vi "Last_Window.vi"(0 "Produced_Time":timestamp[](array[timestamp]), 4 "Windows_Last_Index":i32, 5 "Window_Spark_Rate_IN":dbl[](array[numeric]), 6 "Threshold [uA]":dbl=0.05 min=0.0001 max=50.0 format="%#_13g", 7 "Window_Median_IN":dbl[](array[numeric]), 9 "Window_Avg_IN":dbl[](array[numeric]), 10 "Window size [min]":i64=5 min=1 max=180, 11 "Origin_Time":timestamp[](array[timestamp]), 15 "Origin_Current_IN":dbl[](array[numeric])) -> (1 "Time_Out":timestamp[](array[timestamp]), 3 "Window_Avg_OUT":dbl[](array[numeric]), 8 "Window_Median_OUT":dbl[](array[numeric]), 12 "Last_Window":cluster{timestamp[], dbl[]}(graph), 14 "Window_Spark_Rate_OUT":dbl[](array[numeric]))   [LabVIEW 2018]
uses:
  <vilib>/Analysis/NI_AALBase.lvlib
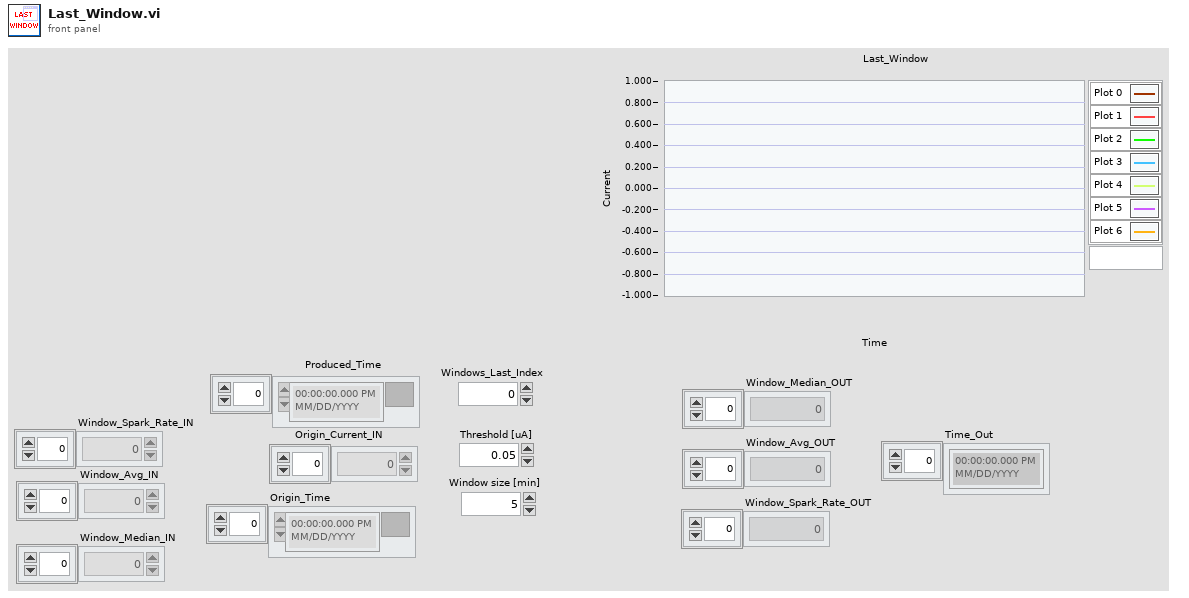
[diagram p1: front panel]
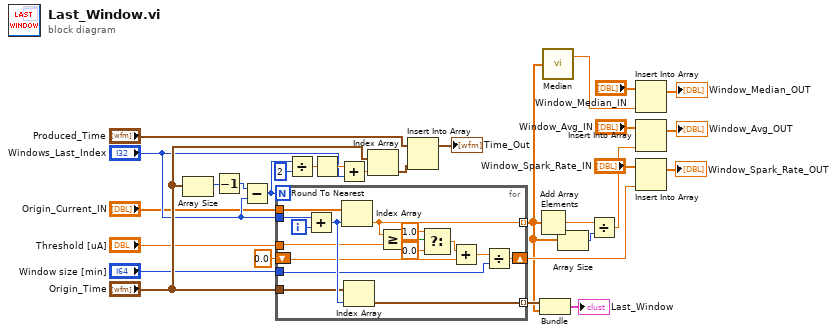
[diagram p0: block diagram]
diagram:
  n1 = Array Size(array="Origin_Time") -> (size(s)=w29:i32)
  n2 = Decrement(x=w29) -> (x-1=w18:i32)
  n3 = Subtract(x=w18, y="Windows_Last_Index") -> (x-y=w25:i32)
  n4 = for {
    N: w25 -> [_]
    tunnel: "Origin_Current_IN" -> [w35]
    tunnel: "Windows_Last_Index" -> [w46]
    tunnel: [w36] -> w2 mode=indexing
    tunnel: "Origin_Time" -> [w43]
    tunnel: [w42] -> w28 mode=indexing
    shift-right: [w34] -> w21
    shift-left: 0.0 -> [w33]
    tunnel: "Threshold [uA]" -> [w32]
    tunnel: "Window size [min]" -> [w31]
    i -> [w45]
    n5 = Add(x=w46, y=w45) -> (x+y=w44:i32)
    n6 = Index Array(array=w35, index=w44) -> (element=w36:dbl)
    n7 = Index Array(array=w43, index=w44) -> (element=w42:timestamp)
    n8 = Greater Or Equal?(x=w36, y=w32) -> (x >= y?=w40:bool)
    n9 = Select(t=1.0, s=w40, f=0.0) -> (s? t:f=w41:dbl)
    n10 = Add(x=w41, y=w33) -> (x+y=w39:dbl)
    n11 = Divide(x=w39, y=w31) -> (x/y=w34:dbl)
  }
  n12 = Divide(x=w25, y=2) -> (x/y=w24:dbl)
  n13 = Round To Nearest(number=w24) -> (nearest integer value=w23:dbl)
  n14 = Add(x=w23, y="Windows_Last_Index") -> (x+y=w22:dbl)
  n15 = Index Array(array="Origin_Time", index=w22) -> (element=w19:timestamp)
  n16 = Insert Into Array(array="Produced_Time", new element=w19) -> (→"Time_Out":timestamp[])  [unwired: 1 in]
  n17 = Add Array Elements(numeric array=w2) -> (sum=w27:dbl)
  n18 = Bundle(w28, w2) -> (→"Last_Window":cluster{timestamp[], dbl[]})  [unwired: 1 in]
  n19 = call <vilib>:"Median.vi"("X"=w2) -> ("median"=w1:dbl)  [unwired: 1 out]
  n20 = Array Size(array=w2) -> (size(s)=w26:i32)
  n21 = Divide(x=w27, y=w26) -> (x/y=w20:dbl)
  n22 = Insert Into Array(array="Window_Median_IN", new element=w1) -> (→"Window_Median_OUT":dbl[])  [unwired: 1 in]
  n23 = Insert Into Array(array="Window_Avg_IN", new element=w20) -> (→"Window_Avg_OUT":dbl[])  [unwired: 1 in]
  n24 = Insert Into Array(array="Window_Spark_Rate_IN", new element=w21) -> (→"Window_Spark_Rate_OUT":dbl[])  [unwired: 1 in]
